vi "customize_channel.vi"() -> (2 "Array - String":string[](array[string]))   [LabVIEW 2024]
panel:
  in  "单位":string
  in  "物理量":string
  in  "确认":bool
  in  "取消":bool
  in  "最大值":dbl=5.0
  in  "最小值":dbl=-5.0
  in  "物理通道":tag="Dev1/ai0"
  in  "function tab":enum32{"original", "polynomial"}(tab)
  in  "c":string
  in  "b":string
  in  "a":string
  in  "Cluster":T1={"Terminal Configuration"=-1, "Min Voltage"=-5.0, "Physical Channel"="Dev1/ai0", "Max Voltage"=5.0, "function"="", "on/off"=FALSE, "物理量"="", "单位"=""} {"Terminal Configuration" items=["default"=-1, "RSE"=10083, "NRSE"=10078, "Differential"=10106, "Pseudodifferential"=12529]}
  # "函数变换"
  # "f(x)=x"
  # "f(x)=ax^2+bx+c"
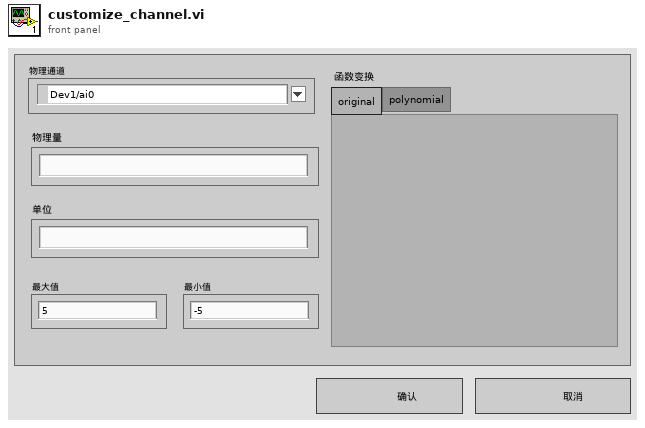
[diagram p1: front panel]
types:
  T1 = cluster{"Terminal Configuration":i32, "Min Voltage":dbl, "Physical Channel":tag, "Max Voltage":dbl, "function":string, "on/off":bool, "物理量":string, "单位":string}
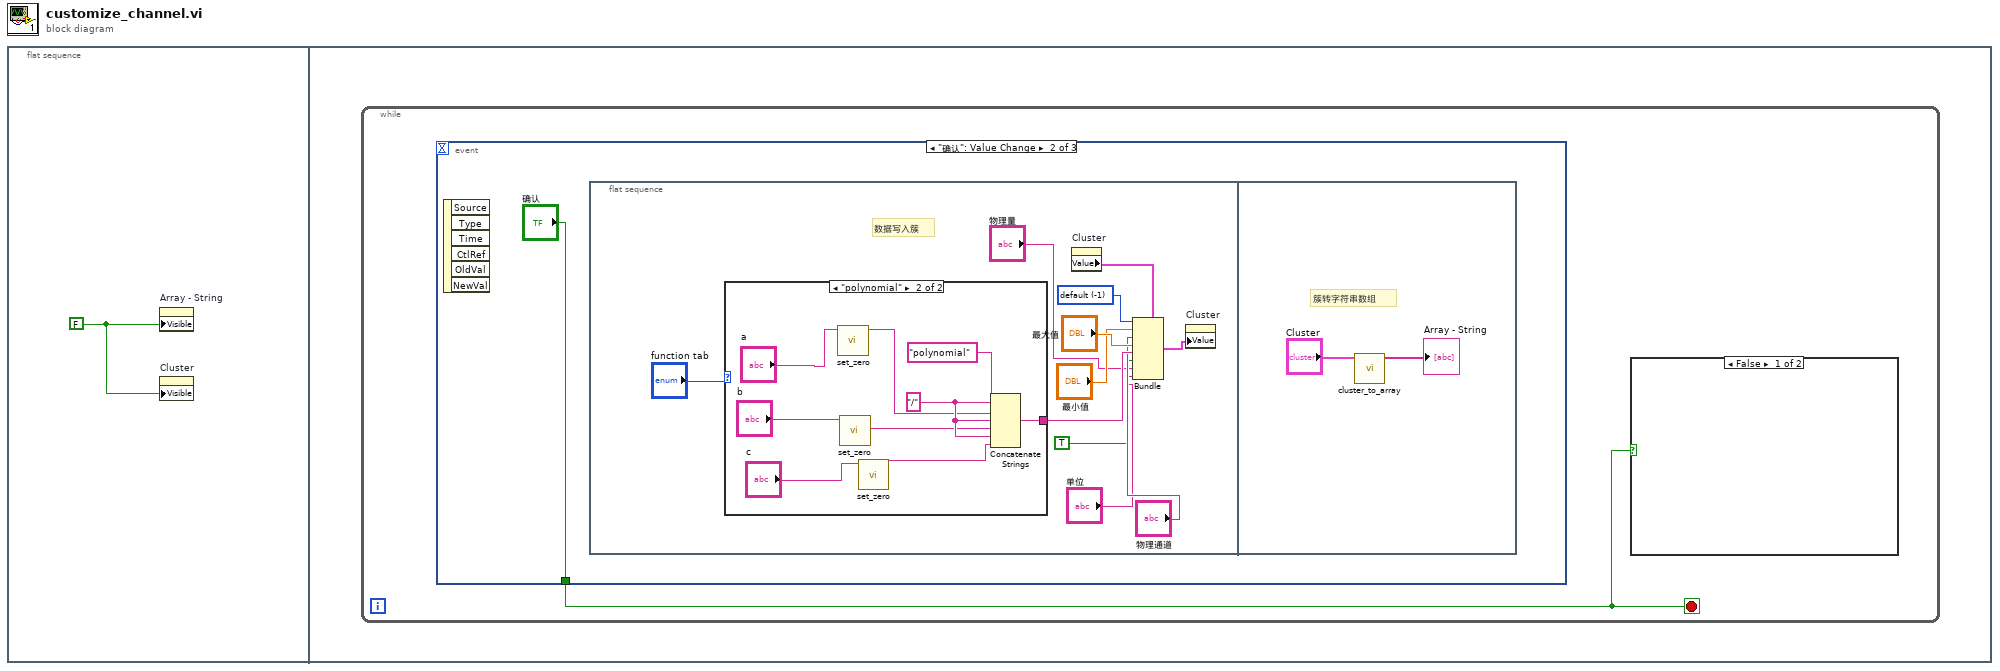
[diagram p0: block diagram]
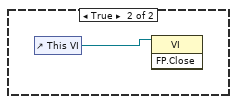
[diagram p2: hidden frame]
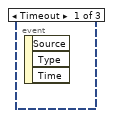
[diagram p3: hidden frame]
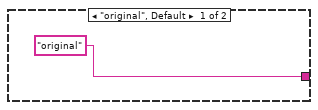
[diagram p4: hidden frame]
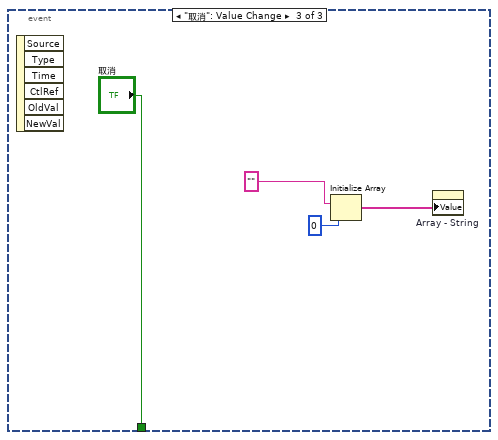
[diagram p5: hidden frame]
diagram:
  n1 = flat-sequence {
    frame #0 {
      w1 = FALSE
      n2 = property on="Array - String" class="Arr (strict)"("Visible"=w1) -> ()  [unwired: 2 in, 2 out]
      n3 = property on="Cluster" class="Clust (strict)"("Visible"=w1) -> ()  [unwired: 2 in, 2 out]
    }
    frame #1 {
      n4 = while {
        stop <- w2 stop-if-true
        n5 = event shown="[1] \"确认\": Value Change" {
          selector: _ -> [_ _ _]
          dyn-events: _ -> [_ _ _]
          timeout: _ -> [_ _ _]
          tunnel: [_ "确认" "取消"] -> w2
          event Timeout {
            n6 = event-data() -> ()  [unwired: 1 in, 3 out]
          }
          event "确认": Value Change {
            n7 = event-data() -> ()  [unwired: 1 in, 6 out]
            n8 = flat-sequence {
              frame #0 {
                w11 = -1 items=["default"=-1, "RSE"=10083, "NRSE"=10078, "Differential"=10106, "Pseudodifferential"=12529] ("Terminal Configuration")
                # "数据写入簇"
                n9 = case shown="\"polynomial\"" "function tab" {
                  tunnel: ["original" w20] -> w12
                  frame "original", Default {
                  }
                  frame "polynomial" {
                    w24 = "/"
                    n10 = call "set_zero.vi"("String in"="a") -> ("String out"=w23:string)  [unwired: 10 in]
                    n11 = call "set_zero.vi"("String in"="b") -> ("String out"=w22:string)  [unwired: 10 in]
                    n12 = call "set_zero.vi"("String in"="c") -> ("String out"=w21:string)  [unwired: 10 in]
                    n13 = Concatenate Strings("polynomial", w24, w23, w24, w22, w24, w21) -> (w20:string)
                  }
                }
                n14 = property on="Cluster" class="Clust (strict)"() -> ("Value"=w13:T1)  [unwired: 2 in, 2 out]
                n15 = Bundle(cluster=w13, "Terminal Configuration"=w11, "Min Voltage"="最小值", "Physical Channel"="物理通道", "Max Voltage"="最大值", "function"=w12, "on/off"=TRUE, "物理量"="物理量", "单位"="单位") -> (w14:T1)
                n16 = property on="Cluster" class="Clust (strict)"("Value"=w14) -> ()  [unwired: 2 in, 2 out]
              }
              frame #1 {
                # "簇转字符串数组"
                n17 = call "cluster_to_array.vi"("Cluster"="Cluster") -> ("Array - String"=→"Array - String":string[])  [unwired: 10 in]
              }
            }
          }
          event "取消": Value Change {
            n18 = event-data() -> ()  [unwired: 1 in, 6 out]
            n19 = Initialize Array("", 0 ("dimension size")) -> (w29:string[])
            n20 = property on="Array - String" class="Arr (strict)"("Value"=w29) -> ()  [unwired: 2 in, 2 out]
          }
        }
        n21 = case shown="False" w2 {
          frame False {
          }
          frame True {
            n22 = control-ref of="This VI"() -> (w3:refnum<vi>)
            n23 = invoke class="VI" method="FP.Close"(reference=w3) -> ()  [unwired: 2 in, 3 out]
          }
        }
      }
    }
  }
